vi "Event-Driven Scenario (Polling Method).vi"() -> ()   [LabVIEW 2012]
panel:
  out "Waveform Graph":dynamicdata(graph)
  in  "Acquire Data":bool
  out "Temperature (deg F)":dbl=32.0
  in  "Temperature (deg C)":dbl
  in  "Time Check":bool
  out "current time":timestamp
  in  "Stop":bool
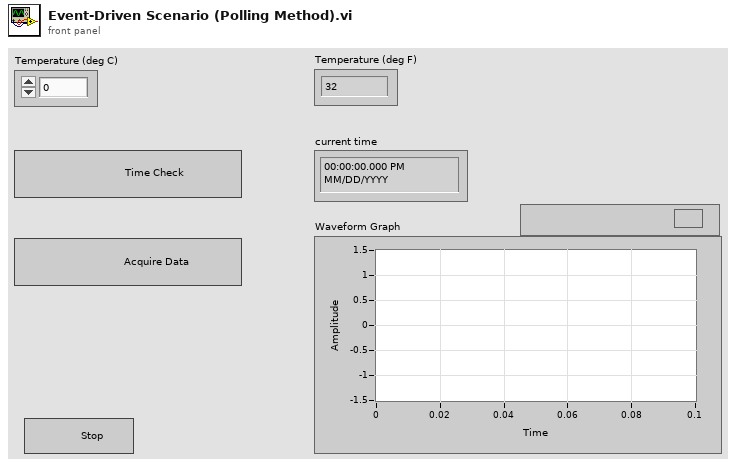
[diagram p1: front panel]
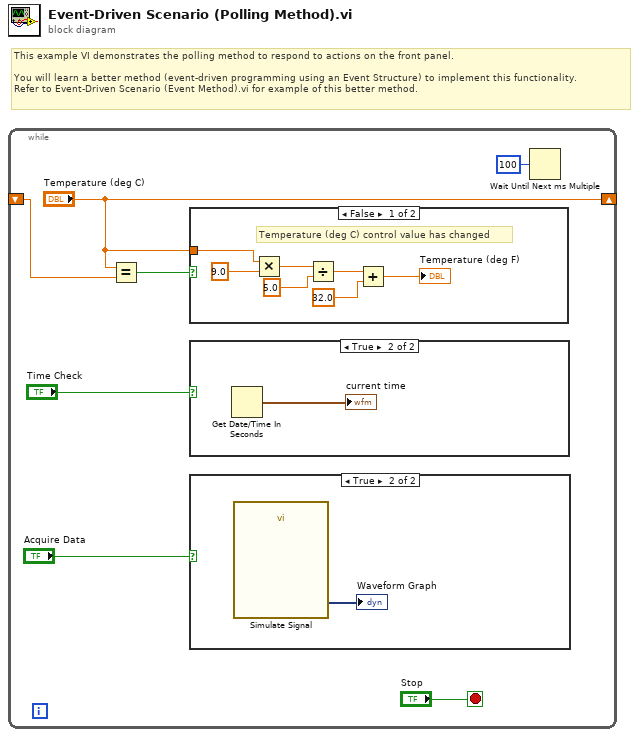
[diagram p0: block diagram]
diagram:
  # "This example VI demonstrates the polling method to respond to actions on the front panel.\n\nYou will learn a better method (event-driven programming using an Event Structure) to implement this functionality.\nRefer to Event-Driven Scenario (Event Method).vi for example of this better method."
  n1 = while {
    shift-right: ["Temperature (deg C)"] -> _
    shift-left: _ -> [w4]
    stop <- "Stop" stop-if-true
    n2 = Equal?(x="Temperature (deg C)", y=w4) -> (x = y?=w3:bool)
    n3 = case shown="False" w3 {
      tunnel: "Temperature (deg C)" -> [w8 _]
      frame False {
        # "Temperature (deg C) control value has changed"
        n4 = Multiply(x=w8, y=9.0) -> (x*y=w13:dbl)
        n5 = Divide(x=w13, y=5.0) -> (x/y=w11:dbl)
        n6 = Add(x=w11, y=32.0) -> (x+y=→"Temperature (deg F)":dbl)
      }
      frame True {
      }
    }
    n7 = case shown="True" "Time Check" {
      frame False {
      }
      frame True {
        n8 = Get Date/Time In Seconds() -> (seconds since 1Jan1904=→"current time":timestamp)
      }
    }
    n9 = case shown="True" "Acquire Data" {
      frame False {
      }
      frame True {
        n10 = call "Simulate Signal"() -> ("Sine with Uniform Noise"=→"Waveform Graph":dynamicdata)  [unwired: 14 in, 1 out]
      }
    }
    n11 = Wait Until Next ms Multiple(millisecond multiple=u32 100) -> ()  [unwired: 1 out]
  }
